vi "testrecycl.vi"() -> ()   [LabVIEW 2019]
uses:
  <vilib>/vision/Instrument.llb/QR Code Report.ctl
  <vilib>/vision/Instrument.llb/QR Code Model Type.ctl
  <vilib>/vision/Instrument.llb/QR Code Stream Mode Type.ctl
  <vilib>/vision/Instrument.llb/Data Matrix Polarity.ctl
  <vilib>/vision/Instrument.llb/Demodulation Mode.ctl
  <vilib>/vision/Instrument.llb/Cell Sample Size.ctl
  <vilib>/vision/Instrument.llb/Cell Filter Mode.ctl
  Global 1.vi
panel:
  in  "Stop (F) in":bool caption="Stop (F)"
  in  "error in (no error)":errorcluster
  out "t":i32
  out "Array":bool[](array[boolean])
  out "appended array":bool[](array[boolean])
  out "Found?":bool
  out "Bounding Box":cluster{"x":sgl, "y":sgl}[](array[cluster])
  out "QR Barcode Report (2D Barcode Reader 1)":T1={"Found?"=FALSE, "Data"="", "Bounding Box"=[], "Errors Corrected"=0, "Dimensions (Rows/Cols)"=0, "Version"=0, "QR Model"=3, "Stream Mode"=0, "Barcode Polarity"=-2, "Mirrored?"=FALSE, "Append Stream Position"=0, "Size of Append Stream"=0, "First EAN-128 ID"=0, "First Alternate Language ID"=0, "Append Stream ID"=0, "Minimum Edge Strength"=30, "Demodulation Mode"=-2, "Cell Sample Size"=-2, "Cell Filter Mode"=-2} {"Append Stream ID" format="%x"; "Cell Filter Mode" items=["Auto-detect"=-2, "Average"=0, "Median"=1, "Central Average"=2, "High Average"=3, "Low Average"=4, "Very High Average"=5, "Very Low Average"=6, "All Filters"=8]; "Cell Sample Size" items=["Auto-detect"=-2, "1x1"=1, "2x2"=2, "3x3"=3, "4x4"=4, "5x5"=5, "6x6"=6, "7x7"=7]; "Demodulation Mode" items=["Auto-detect"=-2, "Histogram"=0, "Local Contrast"=1, "Combination"=2, "All"=3]; "Barcode Polarity" items=["Auto-detect"=-2, "Black on White"=0, "White on Black"=1]; "Stream Mode" items=["Auto-detect", "Numeric", "AlphaNumeric", "Mixed", "Raw Bytes", "UCC/EAN-128 - In Tokens", "UCC/EAN-128 - In Data", "Extended Character Interpretation", "Kanji"]; "QR Model" items=["Auto Detect", "Micro", "Model 1", "Model 2"]; "Version" max=40 step=1}
  in  "Stop (F)":bool
  out "Image Out":T8(plugin-control)
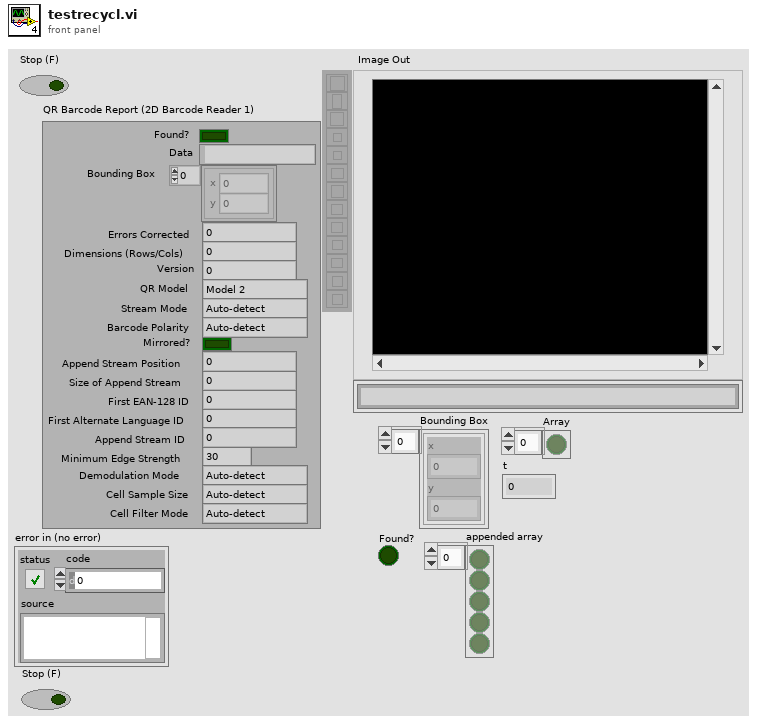
[diagram p1: front panel]
types:
  T1 = typedef "QR Code Report.ctl" = cluster{"Found?":bool, "Data":string, "Bounding Box":cluster{"x":sgl, "y":sgl}[], "Errors Corrected":u32, "Dimensions (Rows/Cols)":u32, "Version":u32, "QR Model":T2, "Stream Mode":T3, "Barcode Polarity":T4, "Mirrored?":bool, "Append Stream Position":u32, "Size of Append Stream":u32, "First EAN-128 ID":i32, "First Alternate Language ID":i32, "Append Stream ID":u32, "Minimum Edge Strength":u32, "Demodulation Mode":T5, "Cell Sample Size":T6, "Cell Filter Mode":T7}
  T2 = typedef "QR Code Model Type.ctl" = i32
  T3 = typedef "QR Code Stream Mode Type.ctl" = i32
  T4 = typedef "Data Matrix Polarity.ctl" = i32
  T5 = typedef "Demodulation Mode.ctl" = i32
  T6 = typedef "Cell Sample Size.ctl" = i32
  T7 = typedef "Cell Filter Mode.ctl" = i32
  T8 = typedef "IMAQ Image.ctl" = refnum<image>
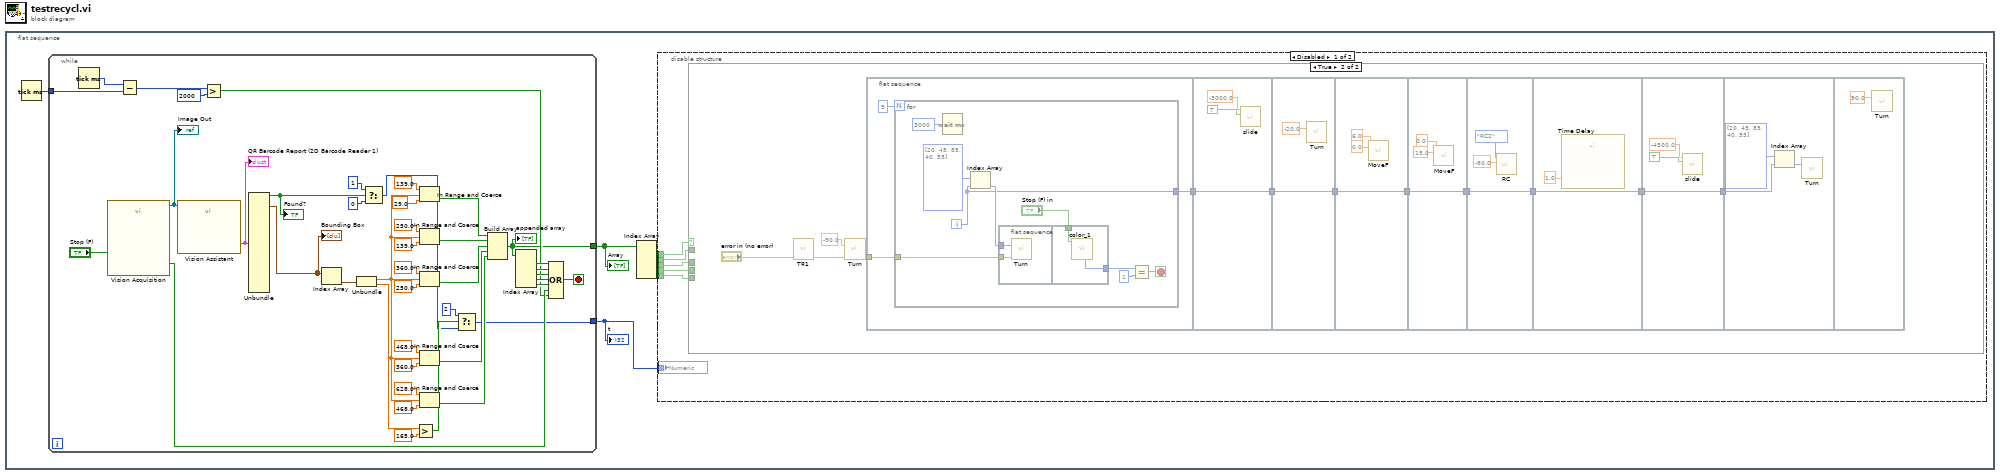
[diagram p0: block diagram]
diagram:
  n1 = flat-sequence {
    frame #0 {
      n2 = Tick Count (ms)() -> (millisecond timer value=w8:u32)
      n3 = while {
        tunnel: w8 -> [w98]
        tunnel: [w87] -> w7
        tunnel: [w78] -> w1
        stop <- w88 stop-if-true
        n4 = Tick Count (ms)() -> (millisecond timer value=w99:u32)
        n5 = call "Vision Acquisition"("Stop (F)"="Stop (F)") -> ("Image Out"=w77:T8, "Stopped"=w90:bool)  [unwired: 24 in, 1 out]
        "Image Out" <- w77
        n6 = Subtract(x=w99, y=w98) -> (x-y=w97:u32)
        n7 = call "Vision Assistant"("Image In"=w77) -> ("QR Barcode Report (2D Barcode Reader 1)"=w76:T1)  [unwired: 24 in, 2 out]
        "QR Barcode Report (2D Barcode Reader 1)" <- w76
        n8 = Greater?(x=w97, y=u32 2000) -> (0:w89:bool)
        n9 = Unbundle(w76) -> ("Found?"=w83:bool, "Bounding Box"=w117:cluster{"x":sgl, "y":sgl}[])  [unwired: 17 out]
        "Bounding Box" <- w117
        "Found?" <- w83
        n10 = Index Array(array=w117) -> (element=w106:cluster{"x":sgl, "y":sgl})  [unwired: 1 in]
        n11 = Unbundle(w106) -> ("x"=w105:sgl, "y"=w86:sgl)
        n12 = Select(t=1, s=w83, f=0) -> (s? t:f=w80:i32)
        n13 = Greater?(x=w86, y=sgl 165.0) -> (0:w84:bool)
        n14 = In Range and Coerce(upper limit=139.0, x=w105, lower limit=29.0) -> (In Range?=w104:bool)  [unwired: 1 out]
        n15 = In Range and Coerce(upper limit=250.0, x=w105, lower limit=139.0) -> (In Range?=w103:bool)  [unwired: 1 out]
        n16 = In Range and Coerce(upper limit=360.0, x=w105, lower limit=250.0) -> (In Range?=w102:bool)  [unwired: 1 out]
        n17 = In Range and Coerce(upper limit=468.0, x=w105, lower limit=360.0) -> (In Range?=w101:bool)  [unwired: 1 out]
        n18 = In Range and Coerce(upper limit=628.0, x=w105, lower limit=468.0) -> (In Range?=w100:bool)  [unwired: 1 out]
        n19 = Select(t=2, s=w84, f=w80) -> (s? t:f=w78:i32)
        n20 = Build Array(w104, w103, w102, w101, w100) -> (w87:bool[])
        "appended array" <- w87
        n21 = Index Array(array=w87) -> (element #1=w95:bool, element #2=w94:bool, element #3=w93:bool, element #4=w92:bool, element #5=w91:bool)  [unwired: 5 in]
        n22 = Compound Arithmetic op=OR(w95, w94, w93, w92, w91, w90, w89) -> (w88:bool)
      }
      "Array" <- w7
      "t" <- w1
      n23 = Index Array(array=w7) -> (element #1=w6:bool, element #2=w5:bool, element #3=w4:bool, element #4=w3:bool, element #5=w2:bool)  [unwired: 5 in]
      n24 = disable-structure shown="Disabled" {
        disable-tunnel: w6 -> [w14 _]
        disable-tunnel: w5 -> [w13 _]
        disable-tunnel: w4 -> [w12 _]
        disable-tunnel: w3 -> [w11 _]
        disable-tunnel: w2 -> [w10 _]
        disable-tunnel: w1 -> [w9 _]
        frame Disabled {
          n25 = global write "Global 1.vi" "Numeric"(w9) -> ()
          n26 = case shown="True" w14 {
            tunnel: w13 -> [w18 _]
            tunnel: w12 -> [w17 _]
            tunnel: w11 -> [w16 _]
            tunnel: w10 -> [w15 _]
            frame False {
              n27 = case shown="False" w18 {
                tunnel: w17 -> [w21 _]
                tunnel: w16 -> [w20 _]
                tunnel: w15 -> [w19 _]
                frame False {
                  n28 = case shown="False" w21 {
                    tunnel: w20 -> [w23 _]
                    tunnel: w19 -> [w22 _]
                    frame False {
                      n29 = case shown="False" w23 {
                        tunnel: w22 -> [w24 _]
                        frame False {
                          n30 = case shown="True" w24 {
                            frame False {
                            }
                            frame True {
                            }
                          }
                        }
                        frame True {
                        }
                      }
                    }
                    frame True {
                    }
                  }
                }
                frame True {
                }
              }
            }
            frame True {
              n31 = call "TR1.vi"("error in (no error)"="error in (no error)") -> ("error out"=w35:errorcluster)  [unwired: 10 in]
              n32 = call "Turn.vi"("角度"=-90.0, "error in (no error)"=w35) -> ("error out"=w33:errorcluster)  [unwired: 13 in]
              n33 = flat-sequence {
                tunnel: w33 -> [w38]
                tunnel: [w37] -> w32
                tunnel: w32 -> [w53]
                tunnel: [w53] -> w31
                tunnel: w31 -> [w57]
                tunnel: [w57] -> w30
                tunnel: w30 -> [w60]
                tunnel: [w60] -> w29
                tunnel: w29 -> [w63]
                tunnel: [w63] -> w28
                tunnel: w28 -> [w66]
                tunnel: [w66] -> w26
                tunnel: w26 -> [w68]
                tunnel: [w68] -> w25
                tunnel: w25 -> [w71]
                tunnel: [w71] -> w27
                tunnel: w27 -> [w74]
                frame #0 {
                  n34 = for {
                    N: 5 -> [_]
                    tunnel: w38 -> [w47]
                    tunnel: [w41] -> w37
                    i -> [w41]
                    stop <- w43 stop-if-true
                    n35 = Wait (ms)(milliseconds to wait=u32 3000) -> ()  [unwired: 1 out]
                    n36 = Index Array(array=i32[] [20, 45, 85, 40, 55], index=w41) -> (element=w46:i32)
                    n37 = flat-sequence {
                      tunnel: w47 -> [w50]
                      tunnel: w46 -> [w49]
                      tunnel: [w52] -> w42
                      tunnel: "Stop (F) in" -> [w51]
                      frame #0 {
                        n38 = call "Turn.vi"("角度"=w49, "error in (no error)"=w50) -> ()  [unwired: 13 in, 1 out]
                      }
                      frame #1 {
                        n39 = call "color_1.vi"("Stop (F) in"=w51) -> ("yellow"=w52:i32)  [unwired: 3 in, 7 out]
                      }
                    }
                    n40 = Equal?(x=w42, y=1) -> (x = y?=w43:bool)
                  }
                }
                frame #1 {
                  n41 = call "slide.vi"("Reset Counter"=TRUE, "Numeric"=-3000.0) -> ()  [unwired: 7 in, 3 out]
                }
                frame #2 {
                  n42 = call "Turn.vi"("角度"=-20.0) -> ()  [unwired: 14 in, 1 out]
                }
                frame #3 {
                  n43 = call "MoveF.vi"("X"=6.0, "Y"=0.0) -> ()  [unwired: 13 in, 1 out]
                }
                frame #4 {
                  n44 = call "MoveF.vi"("X"=0.0, "Y"=15.0) -> ()  [unwired: 13 in, 1 out]
                }
                frame #5 {
                  n45 = call "RC.vi"("數值"=-80.0, "選擇RC"=enum16{"請選擇RC", "RC1", "RC2", "RC3"}."RC2") -> ()  [unwired: 9 in, 1 out]
                }
                frame #6 {
                  n46 = call "Time Delay"("Delay Time (s)"=1.0) -> ()  [unwired: 10 in, 1 out]
                }
                frame #7 {
                  n47 = call "slide.vi"("Reset Counter"=TRUE, "Numeric"=-4500.0) -> ()  [unwired: 7 in, 3 out]
                }
                frame #8 {
                  n48 = Index Array(array=i32[] [20, 45, 85, 40, 55], index=w74) -> (element=w72:i32)
                  n49 = call "Turn.vi"("角度"=w72) -> ()  [unwired: 14 in, 1 out]
                }
                frame #9 {
                  n50 = call "Turn.vi"("角度"=90.0) -> ()  [unwired: 14 in, 1 out]
                }
              }
            }
          }
        }
        frame Enabled {
        }
      }
    }
  }
